vi "TCP_TransmitToGUI.vi"() -> ()   [LabVIEW 2018]
panel:
  in  "stop 2":bool
  out "error out":errorcluster
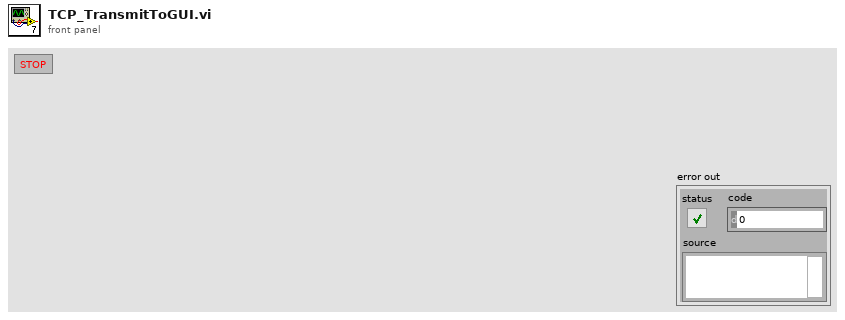
[diagram p1: front panel]
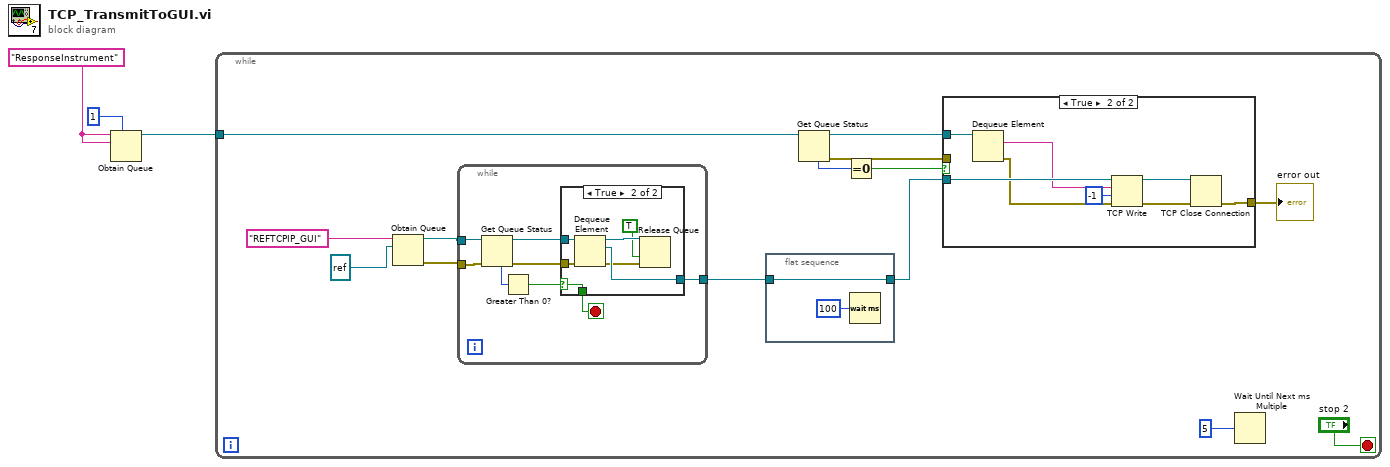
[diagram p0: block diagram]
diagram:
  w3 = "ResponseInstrument"
  n1 = Obtain Queue(max queue size (-1, unlimited)=1, name (unnamed)=w3, element data type=w3) -> (queue out=w2:refnum<queue>)  [unwired: 2 in, 2 out]
  n2 = while {
    tunnel: w2 -> [w16]
    stop <- "stop 2" stop-if-true
    n3 = Obtain Queue(name (unnamed)="REFTCPIP_GUI", element data type=refnum<k5> refnum ("connection ID out")) -> (queue out=w12:refnum<queue>, error out=w11:errorcluster)  [unwired: 3 in, 1 out]
    n4 = while {
      tunnel: [w31] -> w5
      tunnel: w12 -> [w30]
      tunnel: w11 -> [w29]
      stop <- w32 stop-if-true
      n5 = Get Queue Status(queue=w30, error in (no error)=w29) -> (queue out=w36:refnum<queue>, error out=w35:errorcluster, # elements in queue=w33:i32)  [unwired: 1 in, 5 out]
      n6 = Greater Than 0?(x=w33) -> (x > 0?=w34:bool)
      n7 = case shown="True" w34 {
        selector: w34 -> [w37 w42]
        tunnel: w36 -> [_ w44]
        tunnel: w35 -> [_ w43]
        tunnel: [w37 w42] -> w32
        tunnel: [_ w41] -> w31
        frame False {
        }
        frame True {
          n8 = Dequeue Element(queue=w44, error in (no error)=w43) -> (queue out=w40:refnum<queue>, element=w41:refnum<k5>, error out=w39:errorcluster)  [unwired: 1 in, 1 out]
          n9 = Release Queue(queue=w40, force destroy? (F)=TRUE, error in (no error)=w39) -> ()  [unwired: 3 out]
        }
      }
    }
    n10 = flat-sequence {
      tunnel: [w19] -> w4
      tunnel: w5 -> [w19]
      frame #0 {
        n11 = Wait (ms)(milliseconds to wait=u32 100) -> ()  [unwired: 1 out]
      }
    }
    n12 = Get Queue Status(queue=w16) -> (queue out=w8:refnum<queue>, error out=w7:errorcluster, # elements in queue=w10:i32)  [unwired: 2 in, 5 out]
    n13 = Equal To 0?(x=w10) -> (x = 0?=w9:bool)
    n14 = case shown="True" w9 {
      tunnel: w8 -> [_ w28]
      tunnel: w4 -> [_ w27]
      tunnel: w7 -> [w20 _]
      tunnel: [w20 w21] -> w6
      frame False {
      }
      frame True {
        n15 = Dequeue Element(queue=w28) -> (element=w25:string, error out=w24:errorcluster)  [unwired: 2 in, 2 out]
        n16 = TCP Write(connection ID=w27, data in=w25, error in (no error)=w24, 9:-1 ("timeout ms (25000)")) -> (connection ID out=w26:refnum<k5>, error out=w23:errorcluster)  [unwired: 1 out]
        n17 = TCP Close Connection(connection ID=w26, error in (no error)=w23) -> (error out=w21:errorcluster)  [unwired: 1 in, 1 out]
      }
    }
    "error out" <- w6
    n18 = Wait Until Next ms Multiple(millisecond multiple=u32 5) -> ()  [unwired: 1 out]
  }
